vi "Read CtlRef.vi"(8 "error in (no error)":errorcluster, 11 "ControlDragEndedMsg In":refnum<class "ControlDragEndedMsg.lvclass">) -> (0 "error out":errorcluster, 2 "CtlRef":refnum<vi>, 3 "ControlDragEndedMsg Out":refnum<class "ControlDragEndedMsg.lvclass">)   [LabVIEW 2017, in "ActorEvents.lvlib" / "ControlDragEndedMsg.lvclass"]
uses:
  ControlDragEndedMsg.lvclass
  ControlDragEndedMsg.lvclass/ControlDragEndedMsg.ctl
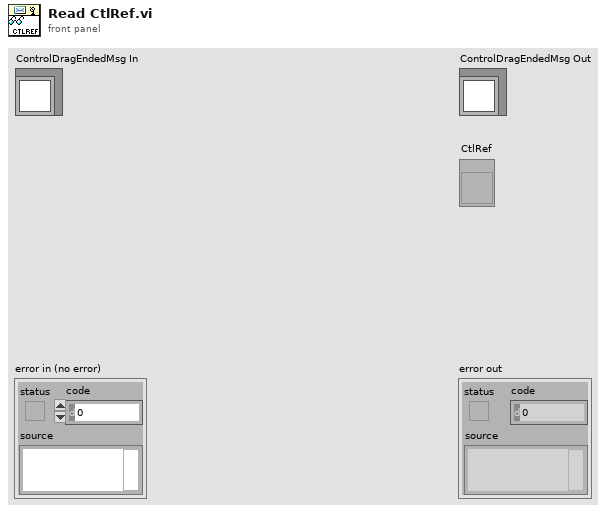
[diagram p1: front panel]
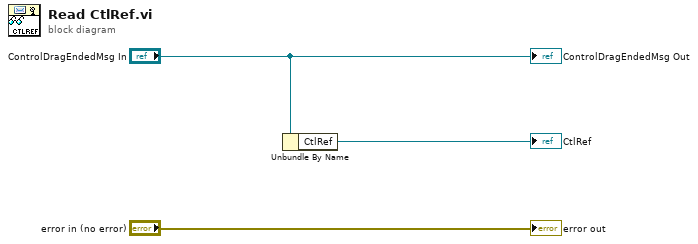
[diagram p0: block diagram]
diagram:
  n1 = Unbundle By Name("ControlDragEndedMsg In") -> ("CtlRef"=→"CtlRef":refnum<vi>)
  "error out" <- "error in (no error)"
  "ControlDragEndedMsg Out" <- "ControlDragEndedMsg In"
